vi "Actor Core.vi"(8 "error in":errorcluster, 11 "Hardware in":refnum<class "pcfs.lvclass">) -> (0 "error out":errorcluster, 3 "Actor out":refnum<class "Actor.lvclass">)   [LabVIEW 2015, in "pcfs.lvclass"]
doc: "(<B>Filename</B>: Actor Framework.lvlib:Actor.lvclass:Actor Core.vi)\n\nReceives messages to the actor, reacts to them, and initiates any error handling that may shut the actor down.\n\nDescendant classes may override this VI to append parallel tasks for the actor to complete while it handles messages. Overrides use the Call Parent Method node."
uses:
  pcfs.lvclass
  <vilib>/ActorFramework/Actor/Actor.lvclass
  Scan/scan_record.ctl
  UI/panel_class/panel.lvclass/panel.ctl
  pcfs_settings.ctl
  Detector_Class/Picoquant/Hydraharp/hydraharp_panel/hpanel_acq_modes.ctl
  <vilib>/ActorFramework/Actor/Actor.lvclass/Actor.ctl
  <vilib>/ActorFramework/Message Enqueuer/Message Enqueuer.lvclass/Message Enqueuer.ctl
  pcfs Messages/pcfs_DO_perform_scan Msg/pcfs_DO_perform_scan Msg.lvclass/pcfs_DO_perform_scan Msg.ctl
  <vilib>/ActorFramework/Message Enqueuer/Init from Existing Queue.vi
  <vilib>/ActorFramework/Message Enqueuer/Enqueue.vi
  custom_trajectories.vi
  <vilib>/ActorFramework/Message Priority Queue/Priority Enqueue.vi
  <vilib>/Analysis/1siggen.llb/Ramp Pattern by Delta.vi
  <vilib>/Utility/file.llb/Read Delimited Spreadsheet (DBL).vi
  <vilib>/ActorFramework/Message Enqueuer/Message Enqueuer.lvclass
  pcfs Messages/pcfs_DO_perform_scan Msg/pcfs_DO_perform_scan Msg.lvclass
  UI/panel_class/panel.lvclass
  <vilib>/Analysis/NI_AALBase.lvlib
panel:
  in  "Path":path
  in  "Custom Path":bool
  in  "File Notes":string
  out "Approx Time":string
  out "Bounds":string
  in  "Cycles":dbl
  in  "Dither Period (s)":dbl
  in  "Dither Dist (nm)":dbl
  in  "Increment (nm)":dbl
  in  "scan":bool
  in  "Record Type":T1
  in  "Save Path":path
  out "Status":string
  in  "Stage Number":enum16{"1", "2"}(ring)
  in  "Steps":dbl
  in  "Center Pos. (mm)":dbl
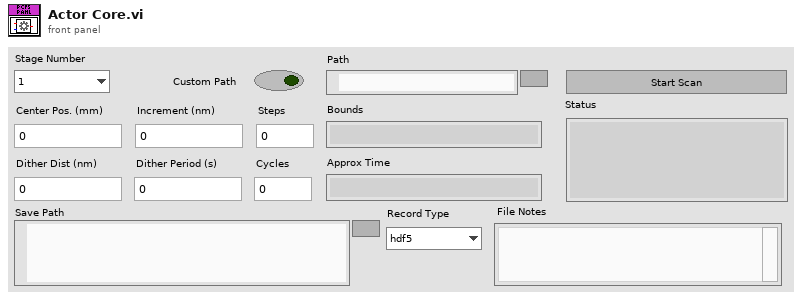
[diagram p1: front panel]
types:
  T1 = typedef "scan_record.ctl" = enum16{"hdf5", "legacy", "None"}
  T2 = cluster{"stop_ui_ref":refnum<event-registration>, "update_status":refnum<event-registration>}
  T3 = typedef "pcfs_settings.ctl" = cluster{"Center Pos. (mm)":dbl, "Increment (mm)":dbl, "Steps":dbl, "Dither Dist (nm)":dbl, "Dither Period (s)":dbl, "Cycles":dbl, "Record Type":T1, "Save Path":path, "Stage Number":enum16{"1", "2"}, "File Notes":string, "Mode":T4, "overwrite":bool, "custom_path":bool, "custom_positions":dbl[]}
  T4 = typedef "hpanel_acq_modes.ctl" = u16
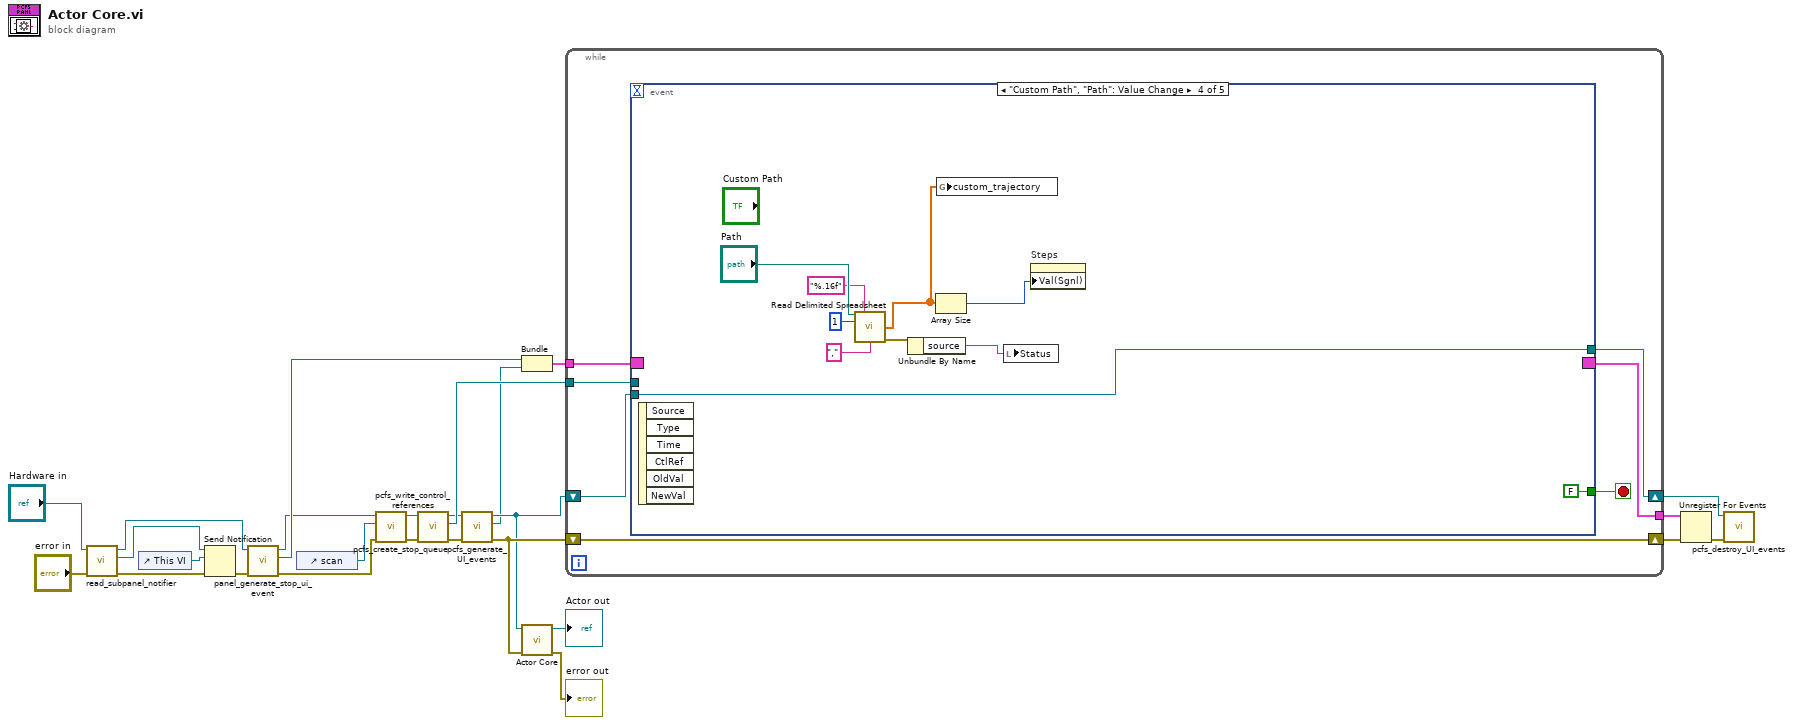
[diagram p0: block diagram]
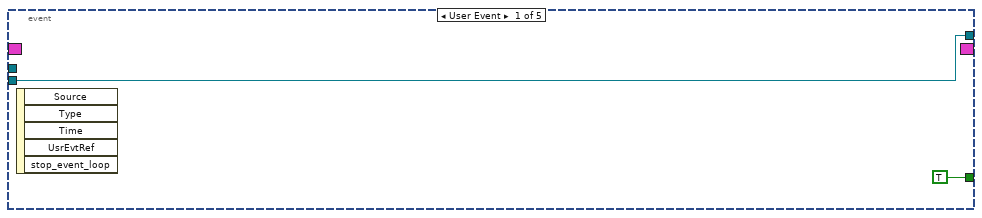
[diagram p2: hidden frame]
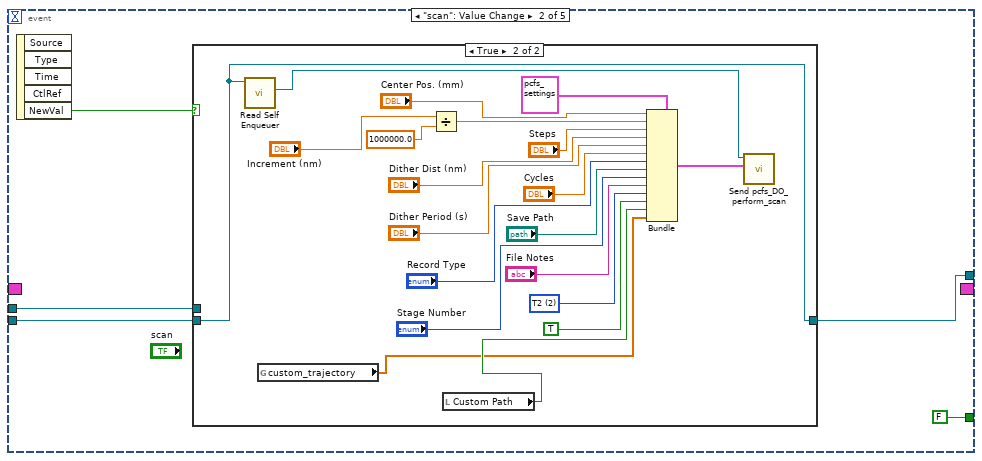
[diagram p3: hidden frame]
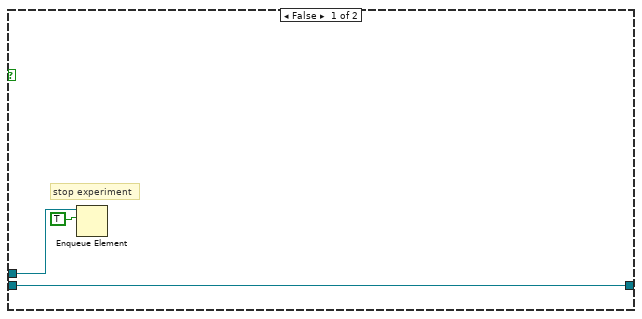
[diagram p4: hidden frame]
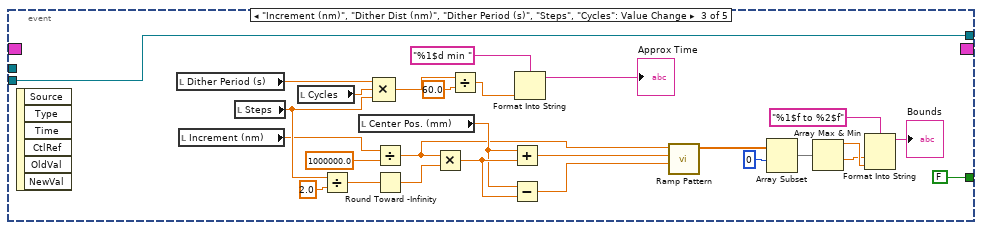
[diagram p5: hidden frame]
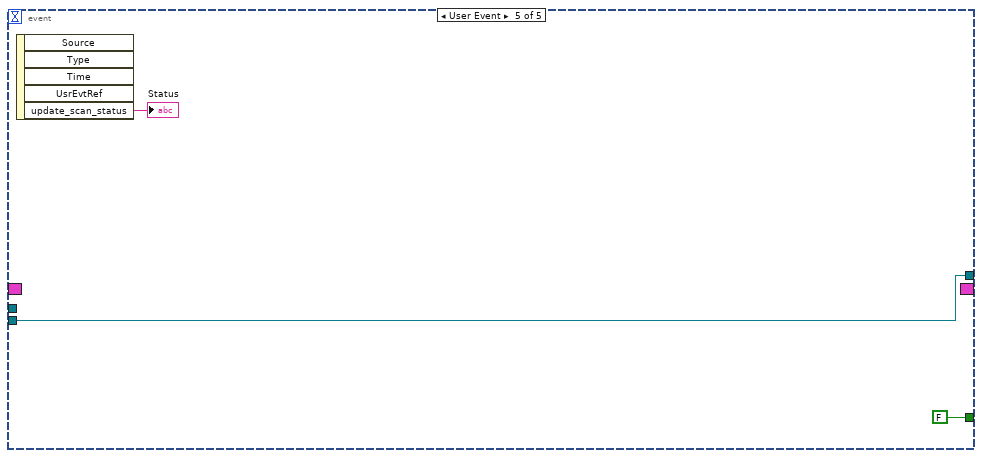
[diagram p6: hidden frame]
diagram:
  n1 = call "read_subpanel_notifier.vi"("error in (no error)"="error in", "panel in"="Hardware in") -> ("error out"=w20:errorcluster, "subpanel_notifier"=w22:refnum<notifier>, "panel out"=w21:refnum<class "pcfs.lvclass">)  [unwired: 7 in]
  n2 = control-ref of="This VI"() -> (w24:refnum<vi>)
  n3 = Send Notification(notification=w24, notifier=w22, error in (no error)=w20) -> (error out=w19:errorcluster)  [unwired: 1 out]
  n4 = call "panel_generate_stop_ui_event.vi"("error in (no error)"=w19, "panel in"=w21) -> ("error out"=w5:errorcluster, "stop_ui_ref"=w11:refnum<event-registration>, "panel out"=w3:refnum<class "pcfs.lvclass">)  [unwired: 7 in]
  n5 = control-ref of="scan"() -> (w1:refnum<vi>)
  n6 = call "pcfs_write_control_references.vi"("error in (no error)"=w5, "scan"=w1, "scan_panel in"=w3) -> ("error out"=w4:errorcluster, "scan_panel out"=w2:refnum<class "pcfs.lvclass">)  [unwired: 7 in]
  n7 = call "pcfs_create_stop_queue.vi"("error in (no error)"=w4, "scan_panel in"=w2) -> ("error out"=w15:errorcluster, "stop_queue"=w16:refnum<queue>, "scan_panel out"=w13:refnum<class "pcfs.lvclass">)  [unwired: 7 in]
  n8 = call "pcfs_generate_UI_events.vi"("error in (no error)"=w15, "scan_panel in"=w13) -> ("error out"=w14:errorcluster, "update_status"=w10:refnum<event-registration>, "scan_panel out"=w12:refnum<class "pcfs.lvclass">)  [unwired: 7 in]
  n9 = Bundle("stop_ui_ref"=w11, "update_status"=w10) -> (w9:T2)  [unwired: 1 in]
  n10 = call-parent "Actor Core.vi"("error in"=w14, "Actor in"=w12) -> ("error out"=→"error out":errorcluster, "Actor out"=→"Actor out":refnum<class "Actor.lvclass">)  [unwired: 8 in]
  n11 = while {
    tunnel: w9 -> [w33]
    tunnel: [w31] -> w17
    shift-right: [w30] -> w8
    shift-left: w14 -> [w30]
    tunnel: w16 -> [w29]
    shift-right: [w27] -> w7
    shift-left: w12 -> [w28]
    stop <- w32 stop-if-true
    n12 = event shown="[3] \"Custom Path\", \"Path\": Value Change" {
      selector: w33 -> [_ _ _ _ _]
      dyn-events: [_ _ _ _ _] -> w31
      timeout: _ -> [_ _ _ _ _]
      tunnel: [TRUE FALSE FALSE FALSE FALSE] -> w32
      tunnel: w29 -> [_ w38 _ _ _]
      tunnel: w28 -> [w34 w37 w90 w100 w101]
      tunnel: [w34 w36 w90 w100 w101] -> w27
      event User Event {
        n13 = event-data() -> ()  [unwired: 1 in, 5 out]
      }
      event "scan": Value Change {
        n14 = event-data() -> ("NewVal"=w39:bool)  [unwired: 1 in, 4 out]
        n15 = case shown="True" w39 {
          tunnel: w38 -> [w43 _]
          tunnel: w37 -> [w41 w63]
          tunnel: [w41 w63] -> w36
          frame False {
            # "stop experiment"
            n16 = Enqueue Element(queue=w43, element=TRUE) -> ()  [unwired: 2 in, 3 out]
          }
          frame True {
            w51 = T4 2 items=["T2"=2, "T3"=3] ("Mode")
            n17 = call <vilib>:"Read Self Enqueuer.vi"("Actor"=w63) -> ("Self Enqueuer"=w61:refnum<class "Message Enqueuer.lvclass">)  [unwired: 10 in]
            n18 = global read "custom_trajectories.vi" "custom_trajectory"() -> (w44:dbl[])
            n19 = Divide(x="Increment (nm)", y=1000000.0) -> (x/y=w47:dbl)
            n20 = local read "Custom Path"() -> (w45:bool)
            n21 = Bundle(cluster=T3 {"Center Pos. (mm)"=0.0, "Increment (mm)"=0.0, "Steps"=0.0, "Dither Dist (nm)"=0.0, "Dither Period (s)"=0.0, "Cycles"=0.0, "Record Type"=enum."hdf5", "Save Path"=path "", "Stage Number"=enum."1", "File Notes"="", "Mode"=2, "overwrite"=FALSE, "custom_path"=FALSE, "custom_positions"=[]} ("scan_position_settings"), "Center Pos. (mm)"="Center Pos. (mm)", "Increment (mm)"=w47, "Steps"="Steps", "Dither Dist (nm)"="Dither Dist (nm)", "Dither Period (s)"="Dither Period (s)", "Cycles"="Cycles", "Record Type"="Record Type", "Save Path"="Save Path", "Stage Number"="Stage Number", "File Notes"="File Notes", "Mode"=w51, "overwrite"=TRUE, "custom_path"=w45, "custom_positions"=w44) -> (w46:T3)
            n22 = call "Send pcfs_DO_perform_scan.vi"("scan_position_settings"=w46, "Message Enqueuer"=w61) -> ()  [unwired: 8 in, 2 out]
          }
        }
      }
      event "Increment (nm)", "Dither Dist (nm)", "Dither Period (s)", "Steps", "Cycles": Value Change {
        n23 = event-data() -> ()  [unwired: 1 in, 6 out]
        n24 = local read "Dither Period (s)"() -> (w74:dbl)
        n25 = local read "Increment (nm)"() -> (w66:dbl)
        n26 = local read "Steps"() -> (w72:dbl)
        n27 = local read "Cycles"() -> (w73:dbl)
        n28 = Divide(x=w72, y=2.0) -> (x/y=w84:dbl)
        n29 = local read "Center Pos. (mm)"() -> (w80:dbl)
        n30 = Compound Arithmetic op=MULTIPLY(w74, w73, w72) -> (w70:dbl)
        n31 = Divide(x=w66, y=1000000.0) -> (x/y=w64:dbl)
        n32 = Round Toward -Infinity(1:w84) -> (0:w83:dbl)
        n33 = Multiply(x=w64, y=w83) -> (x*y=w87:dbl)
        n34 = Divide(x=w70, y=60.0) -> (x/y=w68:dbl)
        n35 = Add(x=w80, y=w87) -> (x+y=w86:dbl)
        n36 = Subtract(x=w80, y=w87) -> (x-y=w85:dbl)
        n37 = Format Into String(format string="%1$d min ", w68) -> (resulting string=→"Approx Time":string)  [unwired: 2 in, 1 out]
        n38 = call-poly <vilib>:"Ramp Pattern.vi"("start"=w85, "end"=w86, "delta"=w64) -> ("Ramp Pattern"=w81:dbl[])  [unwired: 6 in, 2 out]
        n39 = Array Subset(array=w81, index=0) -> (w79:dbl[])  [unwired: 1 in]
        n40 = Array Max & Min(array=w79) -> (max value=w78:dbl, min value=w77:dbl)  [unwired: 2 out]
        n41 = Format Into String(format string="%1$f to %2$f", w77, w78) -> (resulting string=→"Bounds":string)  [unwired: 2 in, 1 out]
      }
      event "Custom Path", "Path": Value Change {
        n42 = event-data() -> ()  [unwired: 1 in, 6 out]
        n43 = call-poly <vilib>:"Read Delimited Spreadsheet.vi"("file path (dialog if empty)"="Path", "format (%.3f)"="%.16f", "number of rows (all:-1)"=1, "delimiter (\\t)"="," ("delimiter (\\t)")) -> ("first row"=w92:dbl[], "error out"=w95:errorcluster)  [unwired: 6 in, 4 out]
        n44 = Unbundle By Name(w95) -> ("source"=w94:string)
        n45 = Array Size(array=w92) -> (size(s)=w93:i32)
        n46 = global write "custom_trajectories.vi" "custom_trajectory"(w92) -> ()
        n47 = local write "Status"(w94) -> ()
        n48 = property on="Steps" class="DigNum (strict)"("Val(Sgnl)"=w93) -> ()  [unwired: 2 in, 2 out]
      }
      event User Event {
        n49 = event-data() -> ("update_scan_status"=→"Status":string)  [unwired: 1 in, 4 out]
      }
    }
  }
  n50 = Unregister For Events(event registration refnum=w17, error in=w8) -> (error out=w6:errorcluster)
  n51 = call "pcfs_destroy_UI_events.vi"("error in (no error)"=w6, "scan_panel in"=w7) -> ()  [unwired: 8 in, 2 out]
